vi "test4-SyncMessageWithError_API.vi"(8 "error in":errorcluster, 11 "TestCase in":refnum<class "testcase-CSMMessage.lvclass">) -> (0 "error out":errorcluster, 3 "TestCase out":refnum<class "testcase-CSMMessage.lvclass">)   [LabVIEW 2017, in "testcase-CSMMessage.lvclass"]
uses:
  testcase-CSMMessage.lvclass
  82a3f3a0-c761-4c70-9aec-dba3e6f930bc.vi
  src/user.lib/_NEVSTOP/Communicable State Machine(CSM)/AdvanceAPI/CSM - Make String Arguments Safe.vi
  src/user.lib/_NEVSTOP/Communicable State Machine(CSM)/AdvanceAPI/CSM - Keywords.vi
  <vilib>/addons/_JKI Toolkits/VI Tester/TestCase.llb/TestCase.lvclass
  src/user.lib/_NEVSTOP/Communicable State Machine(CSM)/Communicable State Machine.lvlib
  C:/Program Files (x86)/National Instruments/LabVIEW 2017/vi.lib/addons/_JKI Toolkits/VI Tester/TestCase.llb/TestCase.lvclass
panel:
  out "LoopCount":i32
  out "concatenated string":string
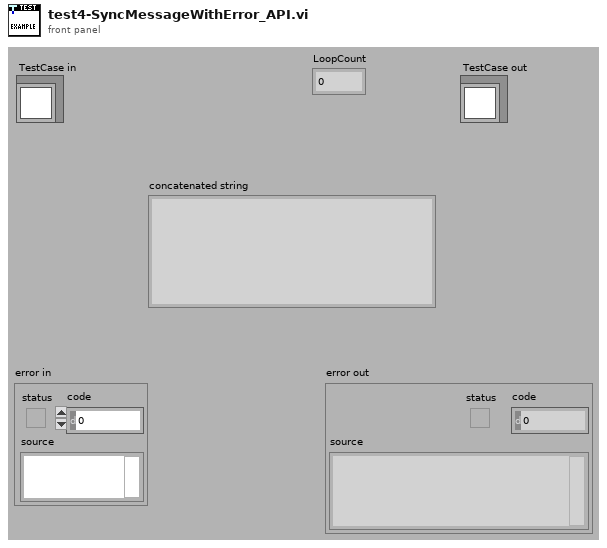
[diagram p1: front panel]
types:
  T1 = cluster{"Arguments":string, "Response":string, "error":errorcluster}
  T2 = cluster{"status":bool, "code":bool, "source":bool}
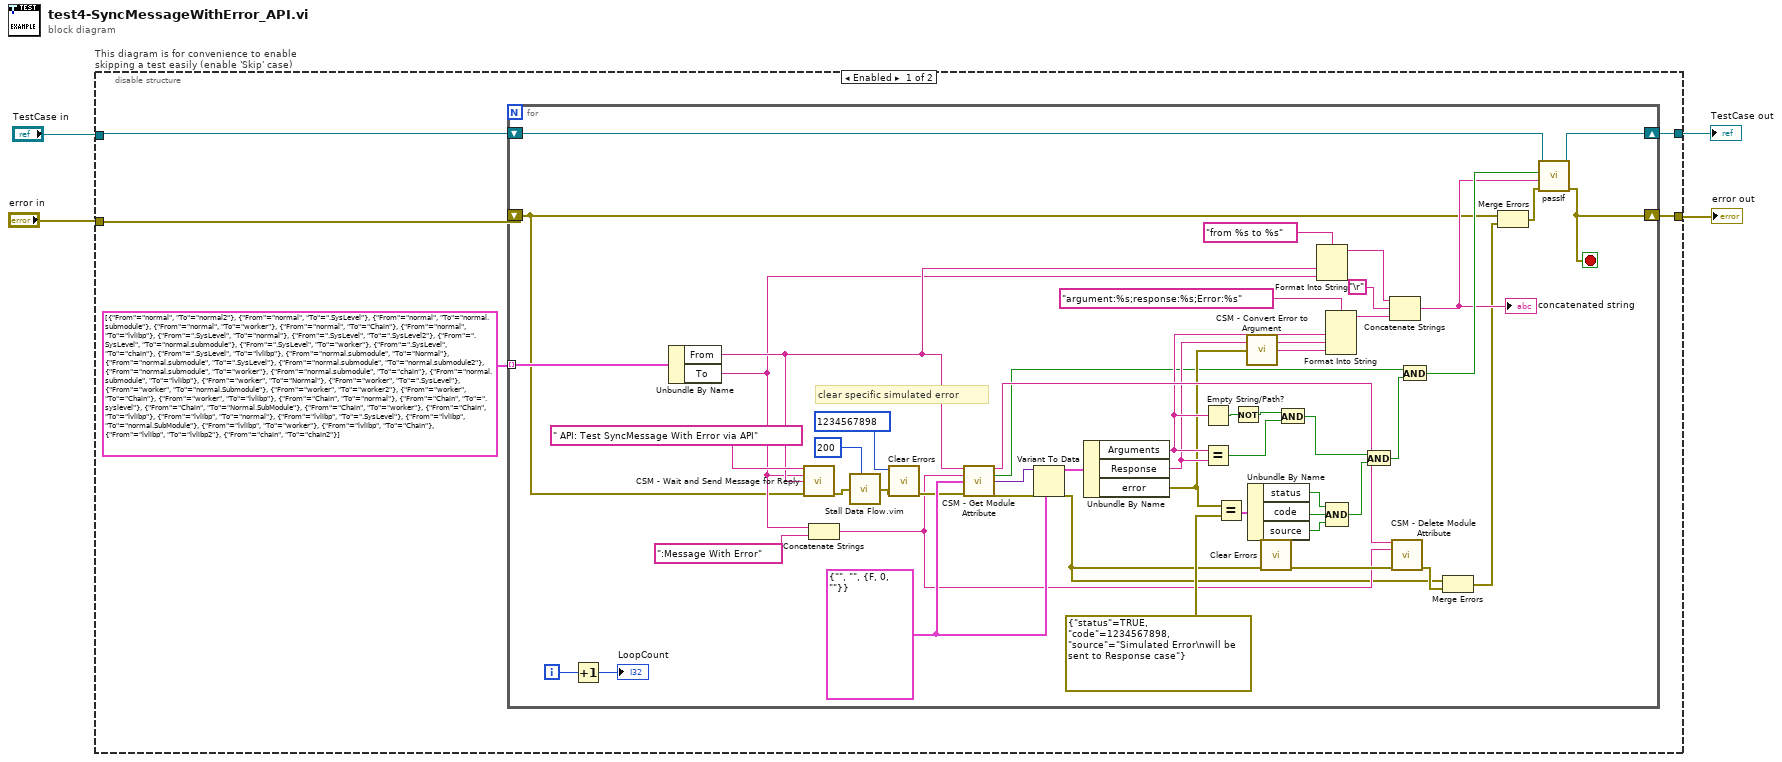
[diagram p0: block diagram]
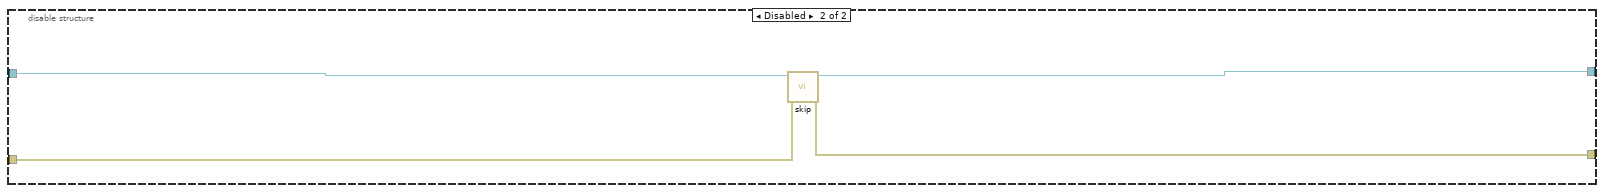
[diagram p2: hidden frame]
diagram:
  n1 = disable-structure "This diagram is for convenience to enable skipping a test easily (enable 'Skip' case)" shown="Enabled" {
    disable-tunnel: "TestCase in" -> [w9 w63]
    disable-tunnel: [w8 w61] -> w1
    disable-tunnel: [w5 w62] -> w3
    disable-tunnel: "error in" -> [w7 w60]
    frame Enabled {
      n2 = for {
        tunnel: cluster{"From":string, "To":string}[] [{"From"="normal", "To"="normal2"}, {"From"="normal", "To"=".SysLevel"}, {"From"="normal", "To"="normal.submodule"}, {"From"="normal", "To"="worker"}, {"From"="normal", "To"="Chain"}, {"From"="normal", "To"="lvlibp"}, {"From"=".SysLevel", "To"="normal"}, {"From"=".SysLevel", "To"=".SysLevel2"}, {"From"=".SysLevel", "To"="normal.submodule"}, {"From"=".SysLevel", "To"="worker"}, {"From"=".SysLevel", "To"="chain"}, {"From"=".SysLevel", "To"="lvlibp"}, {"From"="normal.submodule", "To"="Normal"}, {"From"="normal.submodule", "To"=".SysLevel"}, {"From"="normal.submodule", "To"="normal.submodule2"}, {"From"="normal.submodule", "To"="worker"}, {"From"="normal.submodule", "To"="chain"}, {"From"="normal.submodule", "To"="lvlibp"}, {"From"="worker", "To"="Normal"}, {"From"="worker", "To"=".SysLevel"}, {"From"="worker", "To"="normal.Submodule"}, {"From"="worker", "To"="worker2"}, {"From"="worker", "To"="Chain"}, {"From"="worker", "To"="lvlibp"}, {"From"="Chain", "To"="normal"}, {"From"="Chain", "To"=".syslevel"}, {"From"="Chain", "To"="Normal.SubModule"}, {"From"="Chain", "To"="worker"}, {"From"="Chain", "To"="lvlibp"}, {"From"="lvlibp", "To"="normal"}, {"From"="lvlibp", "To"=".SysLevel"}, {"From"="lvlibp", "To"="normal.SubModule"}, {"From"="lvlibp", "To"="worker"}, {"From"="lvlibp", "To"="Chain"}, {"From"="lvlibp", "To"="lvlibp2"}, {"From"="chain", "To"="chain2"}] -> [w51] mode=indexing
        shift-right: [w58] -> w8
        shift-left: w9 -> [w59]
        shift-right: [w35] -> w5
        shift-left: w7 -> [w14]
        i -> [w17]
        stop <- w35 stop-if-true
        w55 = T1 {"Arguments"="", "Response"="", "error"={"status"=FALSE, "code"=0, "source"=""}}
        # "clear specific simulated error"
        n3 = Increment(x=w17) -> (x+1=→"LoopCount":i32)
        n4 = Unbundle By Name(w51) -> ("From"=w26:string, "To"=w24:string)
        n5 = call "CSM - Wait and Send Message for Reply.vi"("State"=" API: Test SyncMessage With Error via API", "Arguments (\"\")"=w24, "Target Module"=w26, "Error In (No Error)"=w14) -> ("error out"=w22:errorcluster)  [unwired: 8 in, 3 out]
        n6 = Concatenate Strings(w24, ":Message With Error" ("State")) -> (w23:string)
        n7 = call "Stall Data Flow.vim"("value in"=w22, "milliseconds to wait"=u32 200) -> ("value out"=w21:errorcluster)  [unwired: 1 out]
        n8 = call <vilib>:"Clear Errors.vi"("error in (no error)"=w21, "specific error code to clear (0: all)"=1234567898) -> ("error out"=w27:errorcluster)  [unwired: 4 in, 1 out]
        n9 = call "CSM - Get Module Attribute.vi"("CSM Name"=w26, "Attribute"=w23, "Default Value (Empty Variant)"=w55, "Error In"=w27) -> ("CSM Name (Dup)"=w49:string, "Found"=w19:bool, "Value"=w18:variant, "error out"=w56:errorcluster)  [unwired: 7 in, 1 out]
        n10 = Variant To Data(error in=w56, type=w55, Variant=w18) -> (data=w54:T1, error out=w12:errorcluster)
        n11 = Unbundle By Name(w54) -> ("Arguments"=w44:string, "Response"=w43:string, "error"=w34:errorcluster)
        n12 = Empty String/Path?(string/path=w44) -> (empty?=w48:bool)
        n13 = Equal?(x=w44, y=w43) -> (x = y?=w46:bool)
        n14 = Equal?(x=w34, y=errorcluster {"status"=TRUE, "code"=1234567898, "source"="Simulated Error\nwill be sent to Response case"} ("error out")) -> (x = y?=w32:T2)
        n15 = Not(x=w48) -> (.not. x?=w47:bool)
        n16 = call "CSM - Convert Error to Argument.vi"("Error"=w34) -> ("Argument"=w42:string)  [unwired: 4 in]
        n17 = Unbundle By Name(w32) -> ("status"=w31:bool, "code"=w30:bool, "source"=w29:bool)
        n18 = call <vilib>:"Clear Errors.vi"("error in (no error)"=w12) -> ("error out"=w36:errorcluster)  [unwired: 5 in, 1 out]
        n19 = And(x=w47, y=w46) -> (x .and. y?=w45:bool)
        n20 = Format Into String(format string="from %s to %s", w26, w24) -> (resulting string=w38:string)  [unwired: 2 in, 1 out]
        n21 = Format Into String(format string="argument:%s;response:%s;Error:%s", w44, w43, w42) -> (resulting string=w41:string)  [unwired: 2 in, 1 out]
        n22 = Compound Arithmetic op=AND(w31, w30, w29) -> (w28:bool)
        n23 = And(x=w45, y=w28) -> (x .and. y?=w53:bool)
        n24 = Concatenate Strings(w38, "\r", w41) -> (w39:string)
        "concatenated string" <- w39
        n25 = call "CSM - Delete Module Attribute.vi"("CSM Name"=w49, "Attribute"=w23, "Error In"=w36) -> ("error out"=w13:errorcluster)  [unwired: 9 in, 3 out]
        n26 = And(x=w19, y=w53) -> (x .and. y?=w52:bool)
        n27 = Merge Errors(w12, w13) -> (w10:errorcluster)
        n28 = Merge Errors(w14, w10) -> (w11:errorcluster)
        n29 = call-dynamic "passIf.vi"("error in (no error)"=w11, "message (\"\")"=w39, "pass"=w52, "TestCase in"=w59) -> ("error out"=w35:errorcluster, "TestCase out"=w58:refnum<class "testcase-CSMMessage.lvclass">)  [unwired: 6 in]
      }
    }
    frame Disabled {
      # "skip test result while test is under development"
      n30 = call <vilib>:"skip.vi"("error in (no error)"=w60, "TestCase in"=w63) -> ("error out"=w62:errorcluster, "TestCase out"=w61:refnum<class "testcase-CSMMessage.lvclass">)  [unwired: 8 in]
    }
  }
  "error out" <- w3
  "TestCase out" <- w1
